vi "GA_Decode.vi"(6 "Parameters":T1={"Population size"=100, "Generations no."=500, "Significant digits"=4, "Crossover probabality"=0.85, "Mutation mode"=enum."one-point, fixed rate", "Use Gray code?"=FALSE, "Mutation rate"=0.05, "Min mutation rate"=0.0005, "Max mutation rate"=0.25, "Reproduction plan"=enum."Steady-state-replace-worst", "Elitism"=FALSE, "Fmax"=1} {"Max mutation rate" min=0.0 max=1.0; "Min mutation rate" min=0.0 max=1.0; "Mutation rate" min=0.0 max=1.0; "Crossover probabality" min=0.0 max=1.0; "Significant digits" min=1; "Generations no." min=1; "Population size" min=1}, 11 "Genotype":i8[](array[numeric])) -> (3 "Phenotype":i32[](array[numeric]))   [LabVIEW 2016, in "Optimal Frequency Bands Search.lvlib" / "GeneticAlgorithm.lvlib"]
doc: "Преобразовать генотип в фенотип. Возможно кодирование генома с помощью двоичного кода, либо кода Грея"
uses:
  GeneticAlgorithm.lvlib
  GA_tParameters.ctl
panel:
  # "This VI is a part of BCI Design library, http://www.ru-bci.org \nCopyright © 2020, Sotnikov Peter, All rights reserved. License: GNU GPLv3"
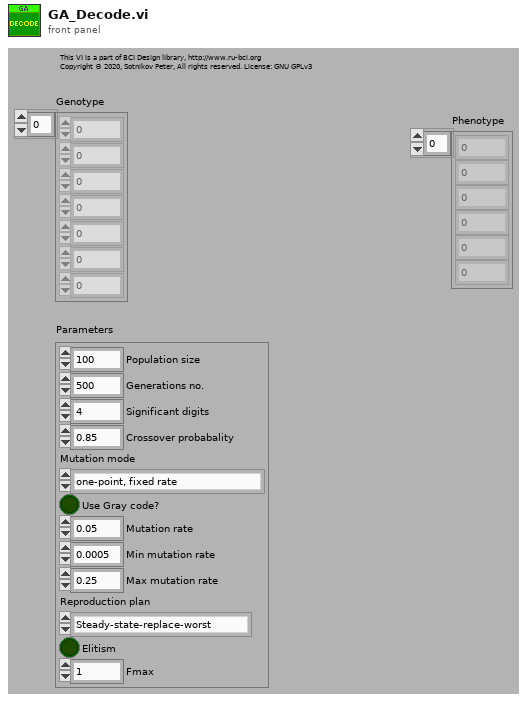
[diagram p1: front panel]
types:
  T1 = typedef "Optimal Frequency Bands Search.lvlib/GeneticAlgorithm.lvlib/GA_tParameters.ctl" = cluster{"Population size":i32, "Generations no.":i32, "Significant digits":i32, "Crossover probabality":dbl, "Mutation mode":enum16{"one-point, fixed rate", "one-point, fitness-adjustable rate", "one-point, distance-adjustable rate"}, "Use Gray code?":bool, "Mutation rate":dbl, "Min mutation rate":dbl, "Max mutation rate":dbl, "Reproduction plan":enum16{"Full generational replacement", "Steady-state-replace-random", "Steady-state-replace-worst"}, "Elitism":bool, "Fmax":i32}
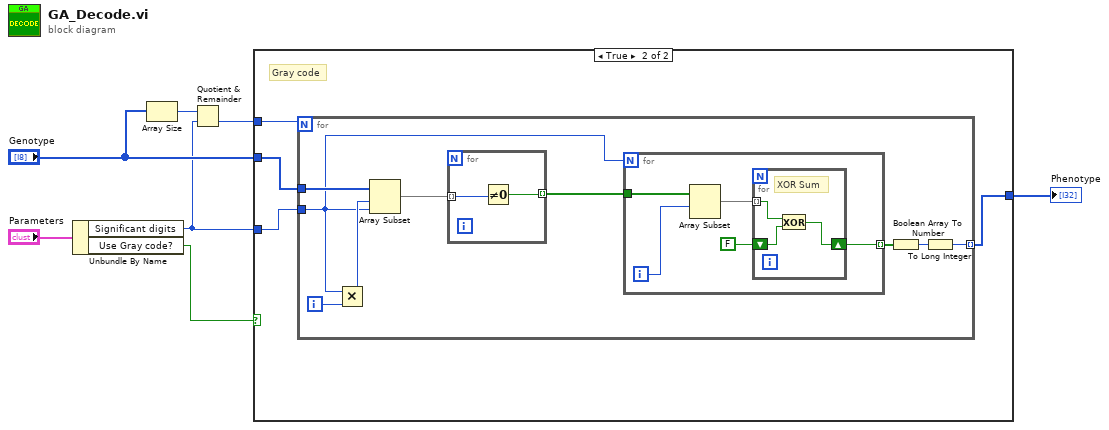
[diagram p0: block diagram]
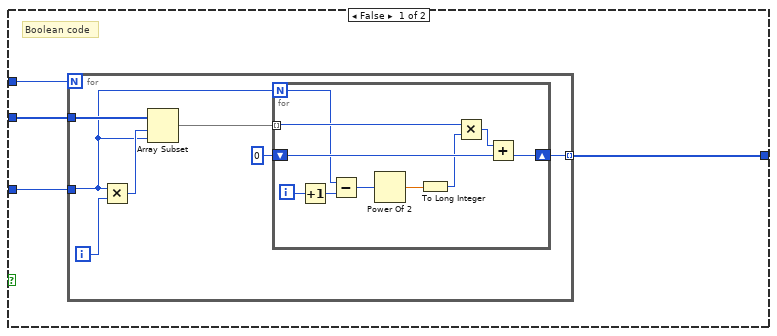
[diagram p2: hidden frame]
diagram:
  n1 = Unbundle By Name("Parameters") -> ("Significant digits"=w3:i32, "Use Gray code?"=w1:bool)
  n2 = Array Size(array="Genotype") -> (size(s)=w7:i32)
  n3 = Quotient & Remainder(x=w7, y=w3) -> (floor(x/y)=w6:i32)  [unwired: 1 out]
  n4 = case shown="True" w1 {
    tunnel: w6 -> [w11 w32]
    tunnel: "Genotype" -> [w10 w31]
    tunnel: w3 -> [w9 w30]
    tunnel: [w8 w29] -> w2
    frame False {
      # "Boolean code"
      n5 = for {
        N: w11 -> [_]
        tunnel: w10 -> [w18]
        tunnel: w9 -> [w13]
        tunnel: [w12] -> w8 mode=indexing
        i -> [w17]
        n6 = Multiply(x=w13, y=w17) -> (x*y=w16:i32)
        n7 = Array Subset(array=w18, index=w16, length=w13) -> (w15:i8[])
        n8 = for {
          N: w13 -> [w24]
          tunnel: w15 -> [w27] mode=indexing
          shift-right: [w28] -> w12
          shift-left: 0 ("x*y") -> [w26]
          i -> [w22]
          n9 = Increment(x=w22) -> (x+1=w23:i32)
          n10 = Subtract(x=w24, y=w23) -> (x-y=w21:i32)
          n11 = Power Of 2(x=w21) -> (2^x=w20:dbl)
          n12 = To Long Integer(number=w20) -> (32bit integer=w19:i32)
          n13 = Multiply(x=w27, y=w19) -> (x*y=w25:i32)
          n14 = Add(x=w25, y=w26) -> (x+y=w28:i32)
        }
      }
    }
    frame True {
      # "Gray code"
      n15 = for {
        N: w32 -> [_]
        tunnel: w31 -> [w41]
        tunnel: w30 -> [w36]
        tunnel: [w33] -> w29 mode=indexing
        i -> [w40]
        n16 = Multiply(x=w36, y=w40) -> (x*y=w39:i32)
        n17 = Array Subset(array=w41, index=w39, length=w36) -> (w38:i8[])
        n18 = for {
          tunnel: w38 -> [w51] mode=indexing
          tunnel: [w50] -> w37 mode=indexing
          n19 = Not Equal To 0?(x=w51) -> (x != 0?=w50:bool)
        }
        n20 = for {
          N: w36 -> [_]
          tunnel: w37 -> [w46]
          tunnel: [w42] -> w35 mode=indexing
          i -> [w45]
          n21 = Array Subset(array=w46, index=w45) -> (w44:bool[])  [unwired: 1 in]
          n22 = for {
            tunnel: w44 -> [w49] mode=indexing
            shift-right: [w47] -> w42
            shift-left: FALSE -> [w48]
            # "XOR Sum"
            n23 = Exclusive Or(1:w48, 2:w49) -> (0:w47:bool)
          }
        }
        n24 = Boolean Array To Number(Boolean array=w35) -> (number=w34:u32)
        n25 = To Long Integer(number=w34) -> (32bit integer=w33:i32)
      }
    }
  }
  "Phenotype" <- w2
